vi "VisObtainQue.vi"(8 "error in (no error)":errorcluster, 10 "QueName":string="BaseVisQue") -> (0 "error out":errorcluster, 3 "queue out":refnum<queue>)   [LabVIEW 2018, in "Visualization.lvlib" / "VisualizeBase.lvclass"]
uses:
  VisualizeBase/VisualizeBase_class/VisualizeBase.lvclass
panel:
  out "created new?":bool
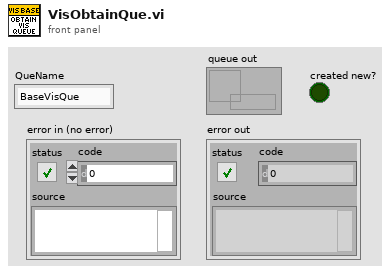
[diagram p1: front panel]
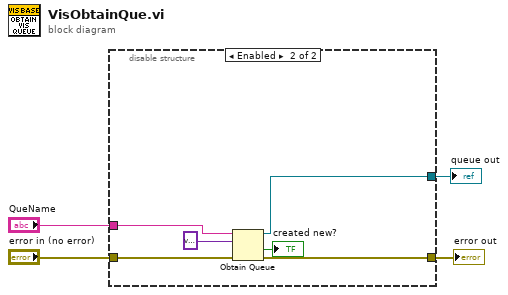
[diagram p0: block diagram]
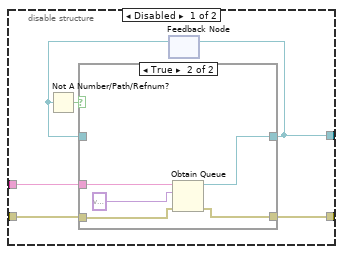
[diagram p2: hidden frame]
diagram:
  n1 = disable-structure shown="Enabled" {
    disable-tunnel: [w10 w19] -> w4
    disable-tunnel: "error in (no error)" -> [w7 w22]
    disable-tunnel: [w6 w21] -> w2
    disable-tunnel: "QueName" -> [w5 w20]
    frame Disabled {
      n2 = feedback #1() -> (w8:refnum<queue>)  [unwired: 1 in]
      n3 = Not A Number/Path/Refnum?(number/path/refnum=w8) -> (NaN/Path/Refnum?=w9:bool)
      n4 = case shown="True" w9 {
        tunnel: [w12 w17] -> w10
        tunnel: w8 -> [w12 _]
        tunnel: w7 -> [w11 w16]
        tunnel: [w11 w15] -> w6
        tunnel: w5 -> [_ w13]
        frame False {
        }
        frame True {
          n5 = Obtain Queue(name (unnamed)=w13, element data type=variant, error in (no error)=w16) -> (queue out=w17:refnum<queue>, error out=w15:errorcluster)  [unwired: 2 in, 1 out]
        }
      }
      n6 = feedback-in #1(w10) -> ()
    }
    frame Enabled {
      n7 = Obtain Queue(name (unnamed)=w20, element data type=variant, error in (no error)=w22) -> (queue out=w19:refnum<queue>, created new?=→"created new?":bool, error out=w21:errorcluster)  [unwired: 2 in]
    }
  }
  "error out" <- w2
  "queue out" <- w4
